vi "DSF.Transceiver.GE Reflective Memory.Transfer to DMA.vi"(8 "error in (no error)":errorcluster, 9 "Transfer in":refnum<class "DSF.Engine.Transfer.lvclass">, 10 "DMA Transfer Spec in":T1 {"Block Descriptors"."descriptor params"."data ptr (lower)" format="%.0x"; "Block Descriptors"."descriptor params"."data ptr (upper)" format="%.0x"; "Block Descriptors"."descriptor params"."data size" format="%.0x"; "Block Descriptors"."descriptor params"."next descriptor ptr" format="%.0x"; "Block Descriptors"."descriptor size" format="%08x"; "Block Descriptors"."descriptor ptr (RFM)" format="%08x"; "Block Descriptors"."descriptor ptr (VISA)" format="%08x"; "RFM offset" format="%08x"}, 11 "GE 5565PIORC in":refnum<class "GE 5565PIORC.lvclass">) -> (0 "error out":errorcluster, 1 "Transfer out":refnum<class "DSF.Engine.Transfer.lvclass">, 2 "DMA Transfer Spec out":T1 {"Block Descriptors"."descriptor params"."data ptr (lower)" format="%.0x"; "Block Descriptors"."descriptor params"."data ptr (upper)" format="%.0x"; "Block Descriptors"."descriptor params"."data size" format="%.0x"; "Block Descriptors"."descriptor params"."next descriptor ptr" format="%.0x"; "Block Descriptors"."descriptor size" format="%08x"; "Block Descriptors"."descriptor ptr (RFM)" format="%08x"; "Block Descriptors"."descriptor ptr (VISA)" format="%08x"; "RFM offset" format="%08x"}, 3 "GE 5565PIORC out":refnum<class "GE 5565PIORC.lvclass">)   [LabVIEW 2017, in "DSF.Transceiver.GE Reflective Memory.lvlib" / "DSF.Transceiver.GE Reflective Memory.lvclass"]
uses:
  DSF.Transceiver.GE Reflective Memory.lvclass
  <vilib>/NI/GE Reflective Memory Driver/GE 5565PIORC.lvclass
  DSF Core/Built/Engine/DSF.Engine.lvlibp/Engine/Classes/Transfer/DSF.Engine.Transfer.lvclass
  DSF Core/Built/Engine/DSF.Engine.lvlibp/Engine/Classes/Buffer/DSF.Engine.Memory.Buffer.lvclass
  <vilib>/NI/GE Reflective Memory Driver/Methods/GE 5565PIORC.DMA.Get Transfer Components (Block).vi
  <vilib>/NI/GE Reflective Memory Driver/Methods/GE 5565PIORC.DMA.Block.Write (Pointer).vi
  <vilib>/NI/GE Reflective Memory Driver/Typedefs/GE 5565PIORC.Typedef.DMA Block Descriptor Params.ctl
  <vilib>/NI/GE Reflective Memory Driver/Typedefs/GE 5565PIORC.Typedef.DMA Block Descriptor.ctl
  <vilib>/NI/GE Reflective Memory Driver/Typedefs/GE 5565PIORC.Typedef.DMA Transfer Spec.ctl
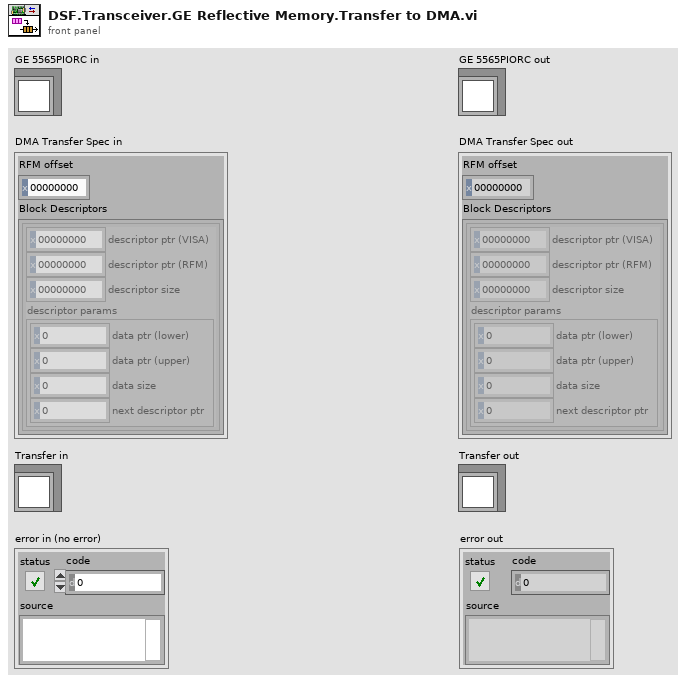
[diagram p1: front panel]
types:
  T1 = typedef "GE 5565PIORC.lvclass/GE 5565PIORC.Typedef.DMA Transfer Spec.ctl" = cluster{"RFM offset":u32, "Block Descriptors":T2[]}
  T2 = typedef "GE 5565PIORC.lvclass/GE 5565PIORC.Typedef.DMA Block Descriptor.ctl" = cluster{"descriptor ptr (VISA)":u32, "descriptor ptr (RFM)":u32, "descriptor size":u32, "descriptor params":T3}
  T3 = typedef "GE 5565PIORC.lvclass/GE 5565PIORC.Typedef.DMA Block Descriptor Params.ctl" = cluster{"data ptr (lower)":u32, "data ptr (upper)":u32, "data size":u32, "next descriptor ptr":u32}
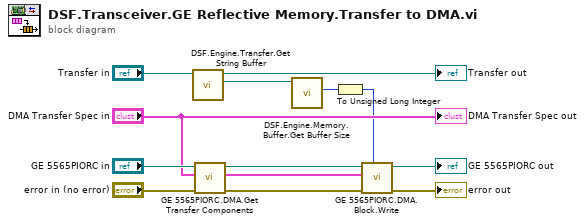
[diagram p0: block diagram]
diagram:
  n1 = call "DSF.Engine.Transfer.Get String Buffer.vi"("Transfer in"="Transfer in") -> ("Buffer"=w10:refnum<class "DSF.Engine.Memory.Buffer.lvclass">, "Transfer out"=→"Transfer out":refnum<class "DSF.Engine.Transfer.lvclass">)  [unwired: 9 in]
  n2 = call-poly <vilib>:"GE 5565PIORC.DMA.Get Transfer Components.vi"("error in (no error)"="error in (no error)", "DMA Transfer Spec in"="DMA Transfer Spec in", "GE 5565PIORC in"="GE 5565PIORC in") -> ("error out"=w6:errorcluster, "Block Descriptor"=w13:T2, "GE 5565PIORC out"=w12:refnum<class "GE 5565PIORC.lvclass">)  [unwired: 5 in, 1 out]
  n3 = call "DSF.Engine.Memory.Buffer.Get Buffer Size.vi"("Buffer in"=w10) -> ("buffer size"=w9:u64)  [unwired: 9 in, 1 out]
  n4 = To Unsigned Long Integer(number=w9) -> (unsigned 32bit integer=w1:u32)
  n5 = call-poly <vilib>:"GE 5565PIORC.DMA.Block.Write.vi"("bytes to move"=w1, "error in (no error)"=w6, "Block Descriptor in"=w13, "GE 5565PIORC in"=w12) -> ("error out"=→"error out":errorcluster, "GE 5565PIORC out"=→"GE 5565PIORC out":refnum<class "GE 5565PIORC.lvclass">)  [unwired: 4 in, 2 out]
  "DMA Transfer Spec out" <- "DMA Transfer Spec in"
